vi "Add Tx Label.vi"(4 "scheduled transmit period (us)":u32=100, 6 "transfer type":T2, 8 "error in":errorcluster, 9 "SDI value":T3=-1 items=["All"=-1, "0 (b00)"=0, "1 (b01)"=1, "2 (b10)"=2, "3 (b11)"=3], 10 "label value":u32, 11 "port ref":T1 format="%.0x") -> (0 "error out":errorcluster, 2 "label":T1 format="%.0x", 3 "port ref out":T1 format="%.0x")   [LabVIEW 2020, in "AIM ARINC 429 Scripting.lvlib"]
doc: "Adds a Tx label to the specified outgoing (Tx) port. Returns the newly added <b>label</b> reference."
uses:
  AIM ARINC 429 Scripting.lvlib
  Constants.vi
  <vilib>/NI VeriStand/Custom Device API/Custom Device API.lvlib
  <vilib>/NI VeriStand/Custom Device API/Custom Device Channel Type.ctl
  <vilib>/NI VeriStand/Custom Device API/Custom Device Channel.ctl
  Shared/Label Properties.ctl
  Shared/Label.ctl
  Import/ARINC 429 Import.lvlib
  <vilib>/NI VeriStand/Custom Device API/Custom Device Item Ref.ctl
  Shared/Transfer Type.ctl
  Shared/SDI.ctl
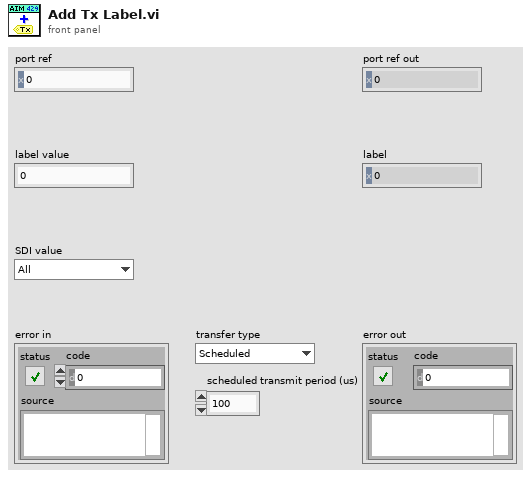
[diagram p1: front panel]
types:
  T1 = typedef "Custom Device API.lvlib/Custom Device Item Ref.ctl" = u64
  T2 = typedef "Transfer Type.ctl" = enum16{"Scheduled", "Acyclic", "Block", "Strobe"}
  T3 = typedef "SDI.ctl" = i32
  T4 = typedef "Direction.ctl" = enum16{"Rx", "Tx"}
  T5 = typedef "Custom Device API.lvlib/Custom Device Channel.ctl" = cluster{"Type":T6, "Units":string, "Default Value":dbl, "Faultable":bool, "Scalable":bool}
  T6 = typedef "Custom Device API.lvlib/Custom Device Channel Type.ctl" = enum16{"Input", "Output"}
  T7 = typedef "Label Properties.ctl" = cluster{"label (Dec)":T8, "SDI value":u8, "SDI enabled":bool}
  T8 = typedef "Label.ctl" = u8
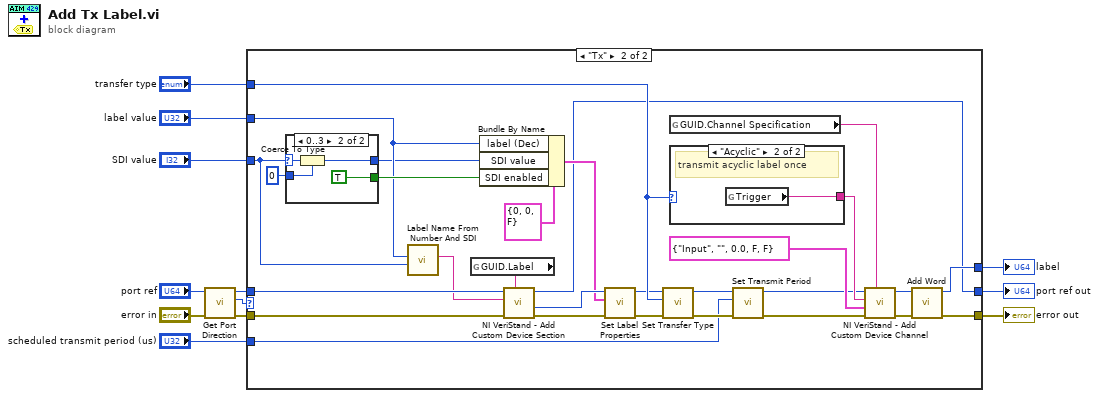
[diagram p0: block diagram]
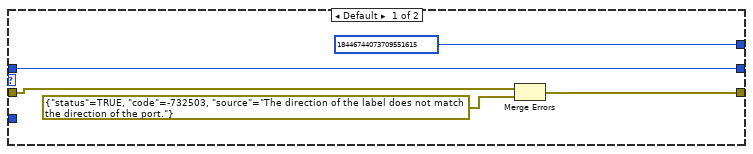
[diagram p2: hidden frame]
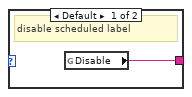
[diagram p3: hidden frame]
diagram:
  n1 = call "Get Port Direction.vi"("error in"="error in", "port ref in"="port ref") -> ("error out"=w8:errorcluster, "direction"=w2:T4, "port ref out"=w9:T1)  [unwired: 7 in]
  n2 = case shown="\"Tx\"" w2 {
    tunnel: [w14 w40] -> w12
    tunnel: w9 -> [w17 w37]
    tunnel: w8 -> [w15 w36]
    tunnel: [T1 18446744073709551615 ("label ref out") w33] -> w7
    tunnel: [w17 w23] -> w6
    tunnel: "transfer type" -> [_ w32]
    tunnel: "label value" -> [_ w29]
    tunnel: "SDI value" -> [_ w27]
    tunnel: "scheduled transmit period (us)" -> [_ w20]
    frame Default {
      n3 = Merge Errors(w15, errorcluster {"status"=TRUE, "code"=-732503, "source"="The direction of the label does not match the direction of the port."} ("error in")) -> (w14:errorcluster)
    }
    frame "Tx" {
      n4 = case shown="0..3" w27 {
        selector: w27 -> [_ w53]
        tunnel: [w49 w50] -> w28
        tunnel: u8 0 ("SDI value") -> [w49 w52]
        tunnel: [_ TRUE] -> w34
        frame Default {
        }
        frame 0..3 {
          n5 = Coerce To Type(0:w53, 1:w52) -> (2:w50:u8)
        }
      }
      n6 = call "Label Name From Number And SDI.vi"("SDI value"=w27, "label (Dec)"=w29) -> ("label name"=w30:string)  [unwired: 9 in]
      n7 = global read "Constants.vi" "GUID.Label"() -> (w41:string)
      n8 = Bundle By Name(cluster=T7 {"label (Dec)"=0, "SDI value"=0, "SDI enabled"=FALSE} ("label properties"), "label (Dec)"=w29, "SDI value"=w28, "SDI enabled"=w34) -> (w38:T7)
      n9 = call <vilib>:"NI VeriStand - Add Custom Device Section.vi"("GUID (Default Section)"=w41, "error in (no error)"=w36, "Section Name"=w30, "Parent Ref in"=w37) -> ("error out"=w43:errorcluster, "Section Ptr"=w42:T1, "Parent Ref out"=w23:T1)  [unwired: 4 in, 1 out]
      n10 = call "Set Label Properties.vi"("error in"=w43, "label properties"=w38, "label ref"=w42) -> ("error out"=w44:errorcluster, "label ref out"=w31:T1)  [unwired: 7 in]
      n11 = call "Set Transfer Type.vi"("error in"=w44, "transfer type"=w32, "label ref in"=w31) -> ("error out"=w22:errorcluster, "label ref out"=w21:T1)  [unwired: 7 in]
      n12 = global read "Constants.vi" "GUID.Channel Specification"() -> (w26:string)
      n13 = case shown="\"Acyclic\"" w32 {
        tunnel: [w47 w48] -> w25
        frame Default {
          # "disable scheduled label"
          n14 = global read "Constants.vi" "Disable"() -> (w47:string)
        }
        frame "Acyclic" {
          # "transmit acyclic label once"
          n15 = global read "Constants.vi" "Trigger"() -> (w48:string)
        }
      }
      n16 = call "Set Transmit Period.vi"("error in"=w22, "transmit period (us)"=w20, "label ref in"=w21) -> ("error out"=w19:errorcluster, "label ref out"=w18:T1)  [unwired: 7 in]
      n17 = call <vilib>:"NI VeriStand - Add Custom Device Channel.vi"("GUID (Default Channel)"=w26, "error in (no error)"=w19, "Channel"=T5 {"Type"=enum."Input", "Units"="", "Default Value"=0.0, "Faultable"=FALSE, "Scalable"=FALSE}, "Channel Name"=w25, "Parent Ref in"=w18) -> ("error out"=w45:errorcluster, "Parent Ref out"=w46:T1)  [unwired: 3 in, 2 out]
      n18 = call "Add Word.vi"("error in"=w45, "label ref"=w46) -> ("error out"=w40:errorcluster, "label ref out"=w33:T1)  [unwired: 6 in, 2 out]
    }
  }
  "label" <- w7
  "error out" <- w12
  "port ref out" <- w6
